vi "GPIO Read.vi"(8 "error in (no error)":errorcluster, 10 "DO Channel":u8, 11 "LINX GPIO in":refnum<class "LINX GPIO.lvclass">) -> (0 "error out":errorcluster, 2 "Input Value":bool, 3 "LINX GPIO out":refnum<class "LINX GPIO.lvclass">)   [LabVIEW 2020, in "LINX GPIO.lvclass"]
uses:
  LINX GPIO.lvclass
  <vilib>/MakerHub/LINX/LMH-LINX.lvlib
  <vilib>/MakerHub/LINX/Public/Peripherals/Digital/Digital Read 1 Chan.vi
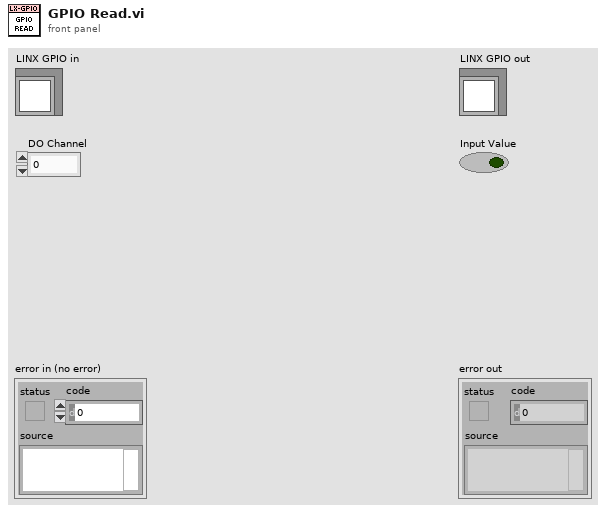
[diagram p1: front panel]
types:
  T1 = typedef "LMH-LINX.lvlib/LINX Ref.ctl" = cluster{"IO":T2, "Interface":T3, "LINX Device Config":T4}
  T2 = typedef "LMH-LINX.lvlib/Platform.ctl" = enum16{"Remote", "Local"}
  T3 = typedef "LMH-LINX.lvlib/Interface.ctl" = enum16{"Serial", "TCP"}
  T4 = typedef "LMH-LINX.lvlib/Device.lvlib/LINX Device Config.ctl" = cluster{"Interface":T3, "COM Port":refnum<visa-resource-name>, "TCP Configuration":T5, "Device Family":u8, "Device ID":u8, "Device Name":string, "TCP Ref":refnum<k5>, "Channels":T6}
  T5 = typedef "LMH-LINX.lvlib/Device.lvlib/TCP Config.ctl" = cluster{"IP Address":string, "Port":u16}
  T6 = typedef "LMH-LINX.lvlib/Channels.ctl" = cluster{"DI":u8[], "DO":u8[], "AI":u8[], "AO":u8[], "PWM":u8[], "QE":u8[], "UART":u8[], "I2C 2":u8[], "SPI":u8[], "CAN":u8[], "Servo":u8[], "AI Ref (V)":dbl, "AI Resolution (Bits)":u8, "AO Ref (V)":dbl, "AO Resolution (Bits)":u8}
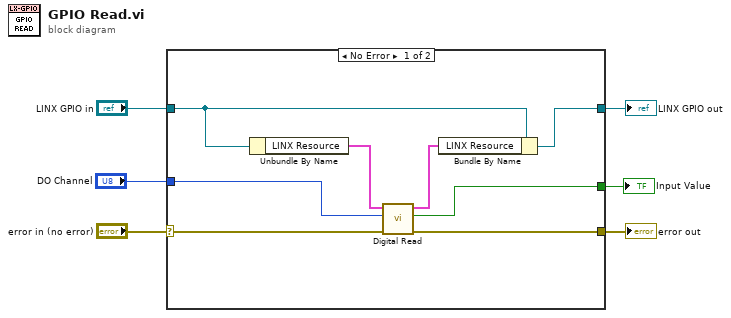
[diagram p0: block diagram]
diagram:
  n1 = case shown="No Error" "error in (no error)" {
    selector: "error in (no error)" -> [w7 w16]
    tunnel: [w8 w16] -> w5
    tunnel: [w13 w15] -> w3
    tunnel: "LINX GPIO in" -> [w14 w15]
    tunnel: "DO Channel" -> [w10 _]
    tunnel: [w9 _] -> w1
    frame No Error {
      n2 = Unbundle By Name(w14) -> ("LINX Resource"=w12:T1)
      n3 = call-poly <vilib>:"Digital Read.vi"("Error In"=w7, "DI Channel"=w10, "LINX Resource"=w12) -> ("Error Out"=w8:errorcluster, "DI Value"=w9:bool, "LINX Resource"=w11:T1)  [unwired: 6 in]
      n4 = Bundle By Name(cluster=w14, "LINX Resource"=w11) -> (w13:refnum<class "LINX GPIO.lvclass">)
    }
    frame Error {
    }
  }
  "error out" <- w5
  "LINX GPIO out" <- w3
  "Input Value" <- w1
